vi "VNA Determine Number of Ports.vi"(9 "Parameter":T1 {"Stimulus Port" min=1 step=1; "Response Port" min=1 step=1}) -> (1 "Number of Ports":i8)   [LabVIEW 2011]
uses:
  tests/S Parameter/TypeDefs/SP Parameter.ctl
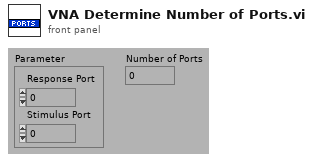
[diagram p1: front panel]
types:
  T1 = typedef "SP Parameter.ctl" = cluster{"Stimulus Port":i8, "Response Port":i8}
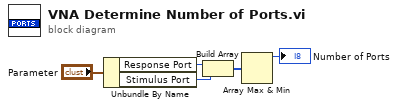
[diagram p0: block diagram]
diagram:
  n1 = Unbundle By Name("Parameter") -> ("Response Port"=w5:i8, "Stimulus Port"=w4:i8)
  n2 = Build Array(w5, w4) -> (w3:i8[])
  n3 = Array Max & Min(array=w3) -> (max value=→"Number of Ports":i8)  [unwired: 3 out]
